vi "Periodic Tasks.vi"(8 "error in":errorcluster) -> ()   [LabVIEW 2011]
doc: "This VI runs in parallel to other tasks. It can contain as many user-defined periodic loops as you need. These can carry out PID or other sorts of timed response."
uses:
  <vilib>/Rock Robotics/SystemInterfaces/Utilities/FPGA_UtilitiesLED State.ctl
  <vilib>/Rock Robotics/SystemInterfaces/Utilities/FPGA_UtilitiesLED Source.ctl
  <vilib>/Rock Robotics/WPI/Relay/WPI_RelayValue.ctl
  Robot Global Data.vi
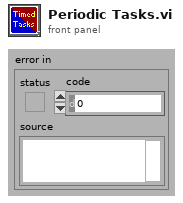
[diagram p1: front panel]
types:
  T1 = typedef "WPI_CompressorDevRef.ctl" = cluster{"DevStatus":errorcluster, "DigitalInputDevRef":T2, "RelayDevRef":T5}
  T2 = typedef "WPI_DigitalInputDevRef.ctl" = cluster{"DevStatus":errorcluster, "DIO Channel":T3, "Digital Module":T4}
  T3 = typedef "FPGA_DIOChannel.ctl" = enum8{"DIO 1", "DIO 2", "DIO 3", "DIO 4", "DIO 5", "DIO 6", "DIO 7", "DIO 8", "DIO 9", "DIO 10", "DIO 11", "DIO 12", "DIO 13", "DIO 14", "Invalid"}
  T4 = typedef "FPGA_TypedefDigitalModule.ctl" = enum16{"Digital Module 1", "Digital Module 2"}
  T5 = typedef "WPI_RelayDevRef.ctl" = cluster{"DevStatus":errorcluster, "Relay Channel":T6, "Digital Module":T4, "Relay Direction":T7}
  T6 = typedef "FPGA_DIORelayChannel.ctl" = enum8{"Relay 1", "Relay 2", "Relay 3", "Relay 4", "Relay 5", "Relay 6", "Relay 7", "Relay 8", "Invalid"}
  T7 = typedef "WPI_RelayDirection.ctl" = enum16{"Both directions", "Forward only", "Reverse only"}
  T8 = typedef "FPGA_UtilitiesLED State.ctl" = enum16{"Off", "On", "Toggle"}
  T9 = typedef "FPGA_UtilitiesLED Source.ctl" = enum16{"User LED", "FPGA LED"}
  T10 = typedef "WPI_EncoderDevRef.ctl" = cluster{"DevStatus":errorcluster, "EncoderIndex":T11, "CounterIndex":T12, "DistancePerCount":dbl, "Decoding Type":T13}
  T11 = typedef "FPGA_EncoderIdx.ctl" = enum8{"Enc 0", "Enc 1", "Enc 2", "Enc 3", "Invalid"}
  T12 = typedef "FPGA_CounterCtrSystemIndex.ctl" = enum8{"Ctr 0", "Ctr 1", "Ctr 2", "Ctr 3", "Ctr 4", "Ctr 5", "Ctr 6", "Ctr 7", "Invalid"}
  T13 = typedef "WPI_EncoderType.ctl" = enum16{"1x", "2x", "4x"}
  T14 = typedef "WPI_RobotDriveDevRef.ctl" = cluster{"DevStatus":errorcluster, "Motors[]":T15[], "Square Inputs":bool, "Max Output":dbl, "Isochronous":bool}
  T15 = typedef "WPI_MotorControlDeviceRef.ctl" = cluster{"DeviceStatus":errorcluster, "Type":enum16{"PWM", "CAN"}, "PWM":cluster{"Digital Module":T4, "PWM Channel":T16, "DeadBand":T17}, "CAN":cluster{"Device Number":u8, "Control Mode":T18, "Semaphore":T19, "Max Vout":dbl}, "Invert":bool, "TransformRef":T20, "InvTransformRef":T20}
  T16 = typedef "FPGA_DIOPWMChannel.ctl" = enum8{"PWM 1", "PWM 2", "PWM 3", "PWM 4", "PWM 5", "PWM 6", "PWM 7", "PWM 8", "PWM 9", "PWM 10", "Invalid"}
  T17 = typedef "WPI_PWMDeadband.ctl" = cluster{"Name":string, "maxPositivePwm":i32, "minPositivePwm":i32, "centerPwm":i32, "maxNegativePwm":i32, "minNegativePwm":i32, "angularRange":u16}
  T18 = typedef "WPI_CANJaguar_ControlMode.ctl" = enum8{"Percent VBus", "Current", "Speed", "Position", "Voltage"}
  T19 = typedef "Semaphore RefNum" = refnum<k1>
  T20 = typedef "WPI_PWMTransform_ConPane.ctl" = refnum<vi>
  T21 = typedef "WPI_JoystickDevRef.ctl" = cluster{"Device":T22}
  T22 = typedef "WPI_JoystickDeviceEnum.ctl" = enum16{"USB 1", "USB 2", "USB 3", "USB 4", "Kinect 1", "Kinect 2"}
  T23 = cluster{"JoystickDevRef":T21, "RobotDriveDevRef":T14}
  T24 = typedef "WPI_GyroDevRef.ctl" = cluster{"DevStatus":errorcluster, "Analog Module":T25, "Analog Channel":T26, "Offset":dbl, "Gain (VoltsPerDegree/Second)":dbl}
  T25 = typedef "FPGA_TypedefAnalogModule.ctl" = enum16{"Analog Module 1", "Analog Module 2"}
  T26 = typedef "FPGA_AIChannel.ctl" = enum8{"AI 1", "AI 2", "AI 3", "AI 4", "AI 5", "AI 6", "AI 7", "AI 8", "Invalid"}
  T27 = typedef "WPI_RelayValue.ctl" = enum16{"Off", "On", "Forward", "Reverse"}
  T28 = cluster{"Digital Input [1-16][0]":bool, "Digital Input [1-16][1]":bool, "Digital Input [1-16][2]":bool, "Digital Input [1-16][3]":bool, "Digital Input [1-16][4]":bool, "Digital Input [1-16][5]":bool, "Digital Input [1-16][6]":bool, "Digital Input [1-16][7]":bool, "Digital Input [1-16][8]":bool}
  T29 = cluster{"axis 1 (x)":dbl, "axis 2 (y)":dbl, "axis 3 (throttle)":dbl, "axis 4":dbl, "axis 5":dbl, "axis 6":dbl}
  T30 = cluster{"Position":cluster{"X":dbl, "Y":dbl}, "Distance (ft)":dbl}[]
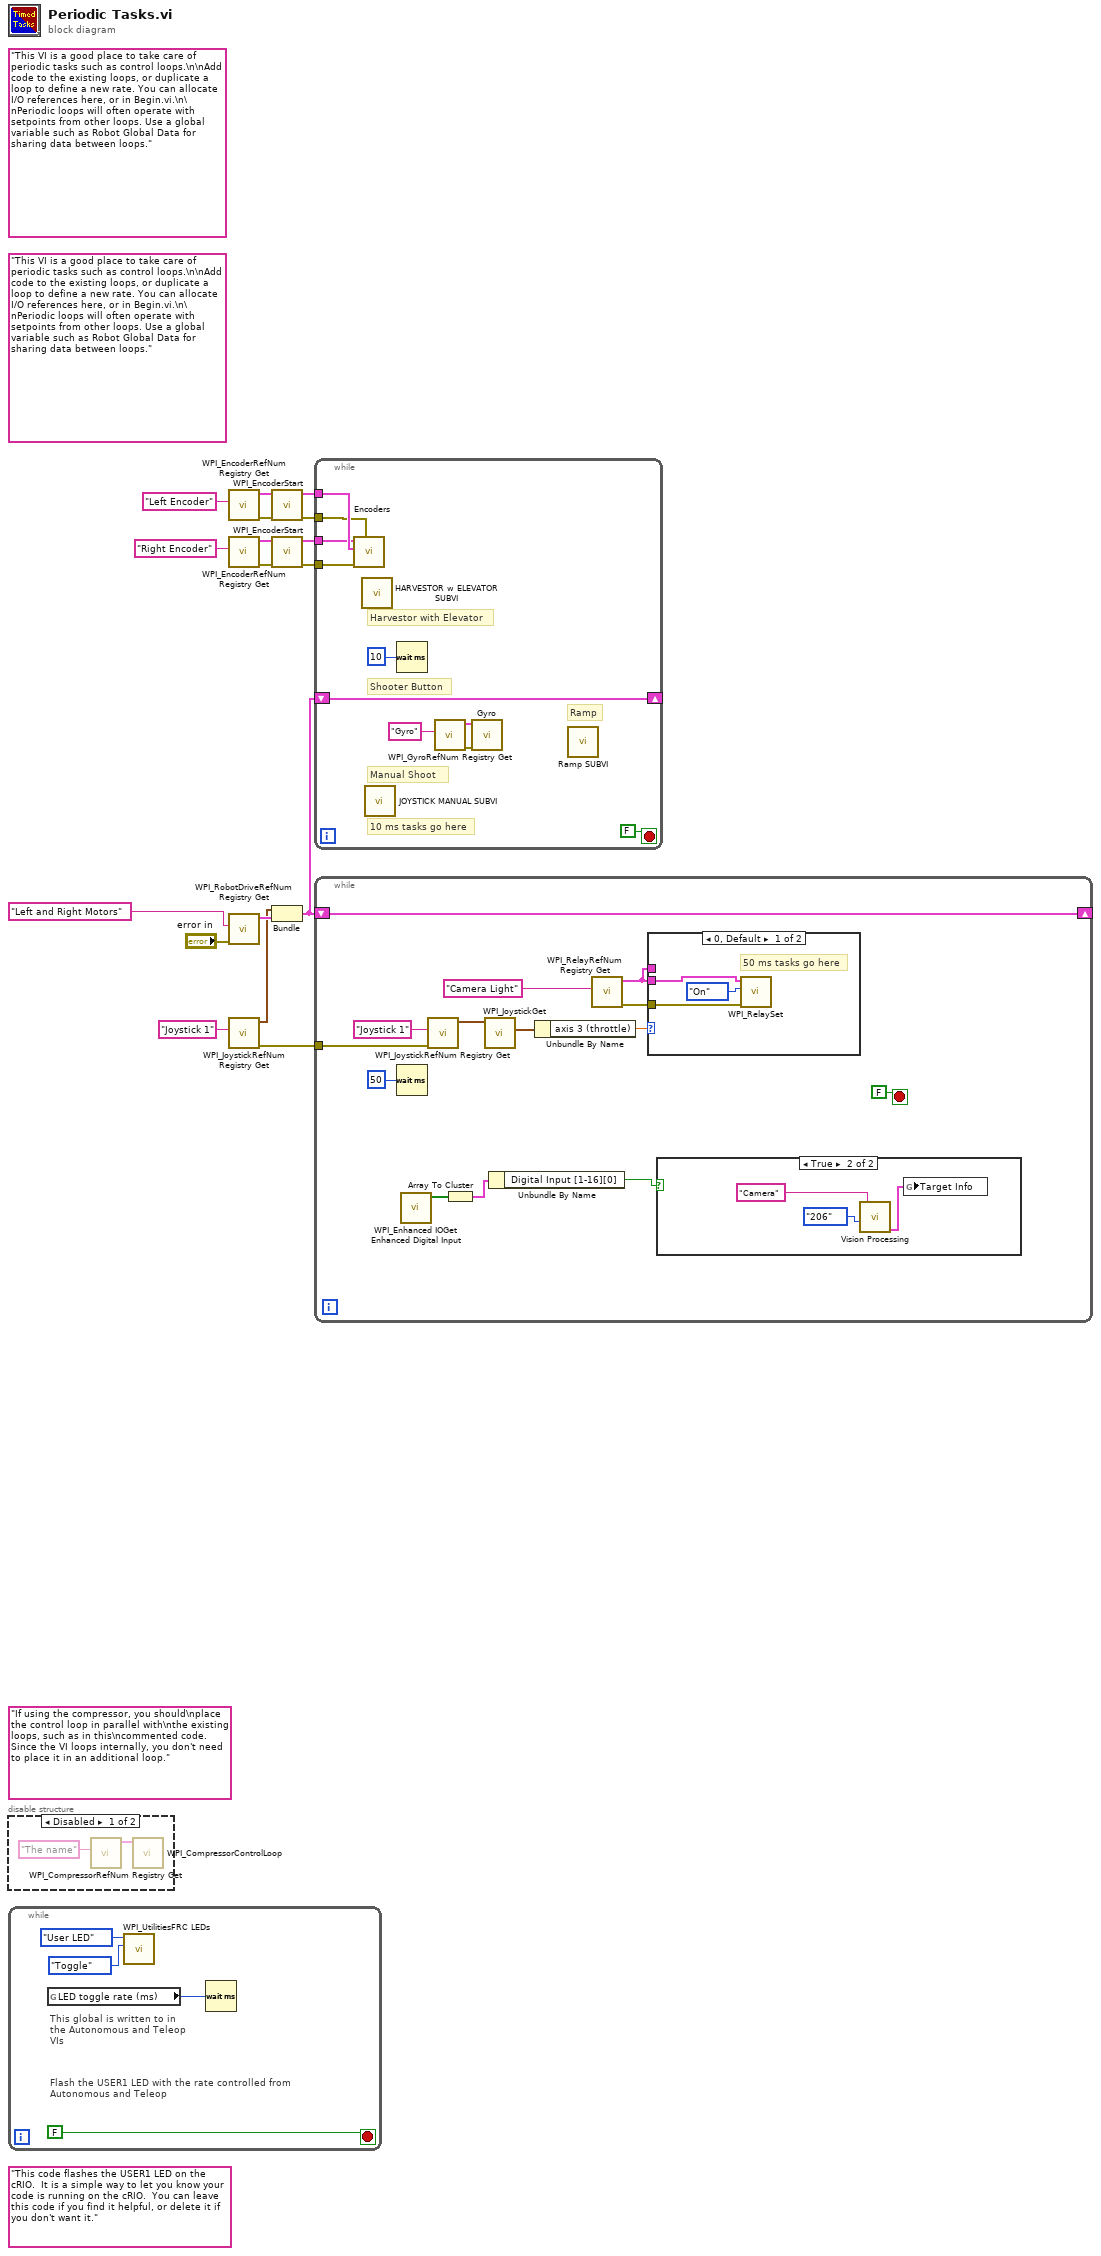
[diagram p0: block diagram]
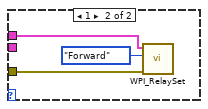
[diagram p4: hidden frame]
diagram:
  (unwired) "This VI is a good place to take care of periodic tasks such as control loops.\n\nAdd code to the existing loops, or duplicate a loop to define a new rate. You can allocate I/O references here, or in Begin.vi.\n\nPeriodic loops will often operate with setpoints from other loops. Use a global variable such as Robot Global Data for sharing data between loops."
  (unwired) "If using the compressor, you should\nplace the control loop in parallel with\nthe existing loops, such as in this\ncommented code. Since the VI loops internally, you don't need to place it in an additional loop."
  (unwired) "This code flashes the USER1 LED on the cRIO.  It is a simple way to let you know your code is running on the cRIO.  You can leave this code if you find it helpful, or delete it if you don't want it."
  (unwired) "This VI is a good place to take care of periodic tasks such as control loops.\n\nAdd code to the existing loops, or duplicate a loop to define a new rate. You can allocate I/O references here, or in Begin.vi.\n\nPeriodic loops will often operate with setpoints from other loops. Use a global variable such as Robot Global Data for sharing data between loops."
  n1 = disable-structure shown="Disabled" {
    frame Disabled {
      n2 = call <vilib>:"WPI_CompressorRefNum Registry Get.vi"("refnum name"="The name") -> ("CompressorDevRef"=w19:T1)  [unwired: 9 in, 1 out]
      n3 = call <vilib>:"WPI_CompressorControlLoop.vi"("CompressorDevRef"=w19) -> ()  [unwired: 11 in]
    }
    frame Enabled {
    }
  }
  n4 = while {
    stop <- FALSE stop-if-true
    # "This global is written to in the Autonomous and Teleop VIs"
    # "Flash the USER1 LED with the rate controlled from Autonomous and Teleop"
    n5 = global read "Robot Global Data.vi" "LED toggle rate (ms)"() -> (w20:u32)
    n6 = call <vilib>:"WPI_UtilitiesFRC LEDs.vi"("State"=FPGA_UtilitiesLED_State."Toggle", "LED Type"=FPGA_UtilitiesLED_Source."User LED") -> ()  [unwired: 1 in, 9 out]
    n7 = Wait (ms)(milliseconds to wait=w20) -> ()  [unwired: 1 out]
  }
  n8 = call <vilib>:"WPI_EncoderRefNum Registry Get.vi"("refnum name"="Left Encoder") -> ("error out"=w6:errorcluster, "EncoderDevRef"=w7:T10)  [unwired: 1 in, 8 out]
  n9 = call <vilib>:"WPI_EncoderRefNum Registry Get.vi"("refnum name"="Right Encoder") -> ("error out"=w9:errorcluster, "EncoderDevRef"=w8:T10)  [unwired: 1 in, 8 out]
  n10 = call <vilib>:"WPI_RobotDriveRefNum Registry Get.vi"("error in (no error)"="error in", "refnum name"="Left and Right Motors") -> ("RobotDriveDevRef"=w15:T14)  [unwired: 9 out]
  n11 = call <vilib>:"WPI_JoystickRefNum Registry Get.vi"("refnum name"="Joystick 1") -> ("error out"=w1:errorcluster, "JoystickDevRef"=w12:T21)  [unwired: 1 in, 8 out]
  n12 = call <vilib>:"WPI_EncoderStart.vi"("error in (no error)"=w6, "EncoderDevRef"=w7) -> ("error out"=w2:errorcluster, "EncoderDevRef"=w5:T10)  [unwired: 8 out]
  n13 = call <vilib>:"WPI_EncoderStart.vi"("error in (no error)"=w9, "EncoderDevRef"=w8) -> ("error out"=w3:errorcluster, "EncoderDevRef"=w4:T10)  [unwired: 8 out]
  n14 = Bundle("JoystickDevRef"=w12, "RobotDriveDevRef"=w15) -> (w14:T23)  [unwired: 1 out]
  n15 = while {
    shift-right: [w31] -> _
    shift-left: w14 -> [w31]
    tunnel: w5 -> [w27]
    tunnel: w4 -> [w26]
    tunnel: w3 -> [w25]
    tunnel: w2 -> [w24]
    stop <- FALSE stop-if-true
    # "Manual Shoot"
    # "Harvestor with Elevator"
    # "Shooter Button"
    # "Ramp"
    # "10 ms tasks go here"
    n16 = call "Encoders.vi"("error in (no error) 2"=w24, "error in (no error)"=w25, "Left Encoder"=w27, "Right Encoder"=w26) -> ()  [unwired: 8 out]
    n17 = call "HARVESTOR w ELEVATOR  SUBVI.vi"() -> ()  [unwired: 12 in]
    n18 = call "JOYSTICK MANUAL SUBVI.vi"() -> ()  [unwired: 12 in]
    n19 = Wait (ms)(milliseconds to wait=u32 10) -> ()  [unwired: 1 out]
    n20 = call <vilib>:"WPI_GyroRefNum Registry Get.vi"("Gyro"="Gyro" ("refnum name")) -> ("error out"=w29:errorcluster, "GyroDevRef"=w28:T24)  [unwired: 1 in, 8 out]
    n21 = call "Gyro.vi"("error in (no error)"=w29, "GyroDevRef"=w28) -> ()  [unwired: 10 out]
    n22 = call "Ramp SUBVI.vi"() -> ()  [unwired: 12 in]
  }
  n23 = while {
    shift-right: [w46] -> _
    shift-left: w14 -> [w46]
    tunnel: w1 -> [w37]
    stop <- FALSE stop-if-true
    n24 = Wait (ms)(milliseconds to wait=u32 50) -> ()  [unwired: 1 out]
    n25 = call <vilib>:"WPI_Enhanced IOGet Enhanced Digital Input.vi"() -> ("Digital Input [1-16]"=w35:bool[])  [unwired: 10 in, 1 out]
    n26 = call <vilib>:"WPI_JoystickRefNum Registry Get.vi"("error in (no error)"=w37, "refnum name"="Joystick 1") -> ("JoystickDevRef"=w40:T21)  [unwired: 8 in, 1 out]
    n27 = Array To Cluster(array=w35) -> (cluster=w36:T28)
    n28 = call <vilib>:"WPI_JoystickGet.vi"("JoystickDevRef"=w40) -> ("Axes"=w43:T29)  [unwired: 4 in, 2 out]
    n29 = Unbundle By Name(w36) -> ("Digital Input [1-16][0]"=w34:bool)
    n30 = Unbundle By Name(w43) -> ("axis 3 (throttle)"=w44:dbl)
    n31 = call <vilib>:"WPI_RelayRefNum Registry Get.vi"("refnum name"="Camera Light") -> ("error out"=w39:errorcluster, "RelayDevRef"=w38:T5)  [unwired: 9 in]
    n32 = case shown="0, Default" w44 {
      tunnel: w39 -> [w52 w54]
      tunnel: w38 -> [w51 _]
      tunnel: w38 -> [_ w55]
      frame 0, Default {
        # "50 ms tasks go here"
        n33 = call <vilib>:"WPI_RelaySet.vi"("error in (no error)"=w52, "RelayValue"=WPI_RelayValue."On", "RelayDevRef"=w51) -> ()  [unwired: 7 in, 2 out]
      }
      frame 1 {
        n34 = call <vilib>:"WPI_RelaySet.vi"("error in (no error)"=w54, "RelayValue"=WPI_RelayValue."Forward", "RelayDevRef"=w55) -> ()  [unwired: 7 in, 2 out]
      }
    }
    n35 = case shown="True" w34 {
      frame False {
      }
      frame True {
        n36 = call "Vision Processing.vi"("Camera Type"=enum16{"206", "1011"}."206", "Camera Name"="Camera") -> ("Target Info"=w48:T30)  [unwired: 2 in, 3 out]
        n37 = global write "Robot Global Data.vi" "Target Info"(w48) -> ()
      }
    }
  }
